vi "Set Enable State on Multiple Controls.vi"(10 "启用？":bool, 11 "控件":refnum<vi>[](array[refnum])) -> ()   [LabVIEW 2014]
doc: "将输入数组中所有控件的值设置为“启用状态”。"
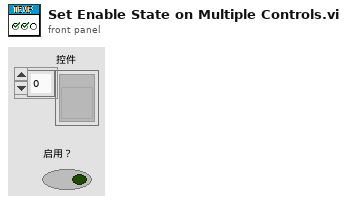
[diagram p1: front panel]
types:
  T1 = enum8{"Enabled", "Disabled", "Disabled and Grayed Out"}
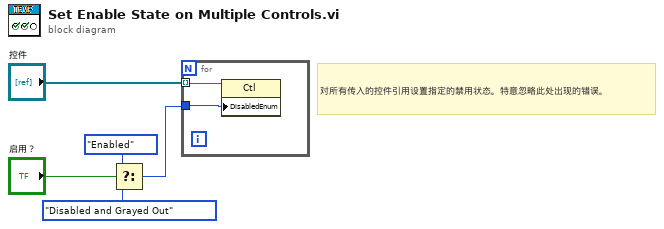
[diagram p0: block diagram]
diagram:
  # "对所有传入的控件引用设置指定的禁用状态。特意忽略此处出现的错误。"
  n1 = Select(t=T1."Enabled" ("Disabled"), s="启用？", f=T1."Disabled and Grayed Out" ("Disabled")) -> (s? t:f=w3:T1)
  n2 = for {
    tunnel: "控件" -> [w7] mode=indexing
    tunnel: w3 -> [w6]
    n3 = property class="Ctl"(reference=w7, "DisabledEnum"=w6) -> ()  [unwired: 1 in, 2 out]
  }
